vi "Init System.vi"(8 "error in (no error)":errorcluster, 11 "Linux System SAL in":refnum<class "Linux System SAL.lvclass">) -> (0 "error out":errorcluster, 3 "Linux System SAL out":refnum<class "Linux System SAL.lvclass">)   [LabVIEW 2020, in "Volatus.lvlib" / "Linux System SAL.lvclass"]
uses:
  Linux System SAL.lvclass
  Linux System SAL.lvclass/Linux System SAL.ctl
  <vilib>/nisyscfg/nisyscfg.lvlib
  <resource>/objmgr/nisysapi.rc
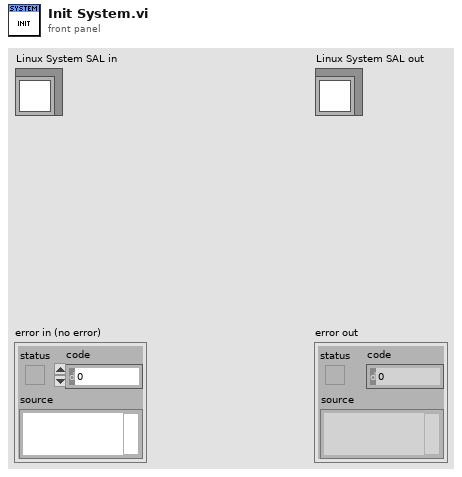
[diagram p1: front panel]
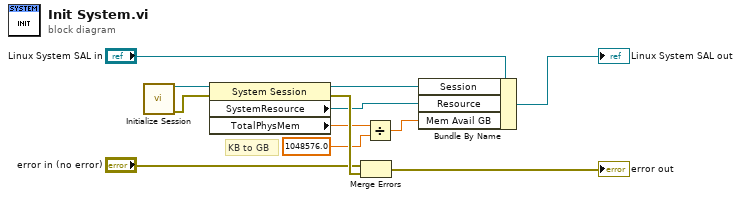
[diagram p0: block diagram]
diagram:
  # "KB to GB"
  n1 = call <vilib>:"Initialize Session.vi"() -> ("error out"=w10:errorcluster, "Session out"=w11:refnum<k21>)  [unwired: 10 in]
  n2 = property class="System Session"(reference=w11, error in=w10) -> (reference out=w9:refnum<k21>, error out=w12:errorcluster, "SystemResource"=w8:refnum<k20>, "TotalPhysMem"=w7:dbl)
  n3 = Merge Errors("error in (no error)", w12) -> (→"error out":errorcluster)
  n4 = Divide(x=w7, y=1048576.0) -> (x/y=w5:dbl)
  n5 = Bundle By Name(cluster="Linux System SAL in", "Session"=w9, "Resource"=w8, "Mem Avail GB"=w5) -> (→"Linux System SAL out":refnum<class "Linux System SAL.lvclass">)
